vi "Send.vi"(8 "error in (no error)":errorcluster, 10 "Message":refnum<class "BaseMessage.lvclass">, 11 "QueueReader in":refnum<class "QueueReader.lvclass">) -> (0 "error out":errorcluster, 2 "Sent Message":refnum<class "BaseMessage.lvclass">, 3 "QueueReader out":refnum<class "QueueReader.lvclass">)   [LabVIEW 2013, in "QueueReader.lvclass"]
doc: "Send a message to the remote destination"
uses:
  QueueReader.lvclass
  Message/BaseMessage/BaseMessage.lvclass
  BaseReader/BaseReader.lvclass
  QueueReader.lvclass/QueueReader.ctl
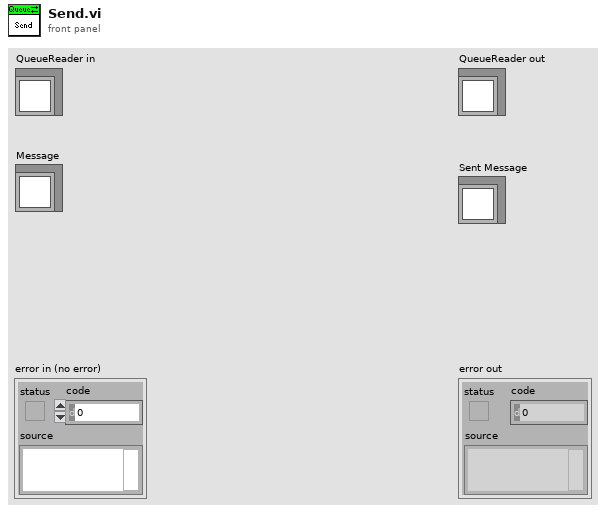
[diagram p1: front panel]
types:
  T1 = typedef "message_queue.ctl" = refnum<queue>
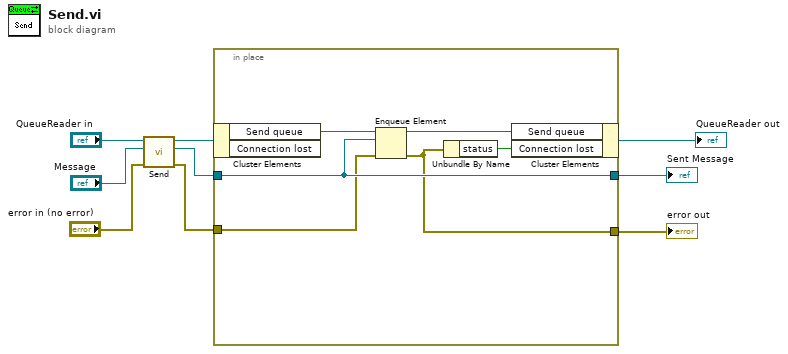
[diagram p0: block diagram]
diagram:
  n1 = call-parent "Send.vi"("error in (no error)"="error in (no error)", "Message"="Message", "BaseReader in"="QueueReader in") -> ("error out"=w1:errorcluster, "Sent Message"=w3:refnum<class "BaseMessage.lvclass">, "BaseReader out"=w5:refnum<class "QueueReader.lvclass">)  [unwired: 6 in]
  n2 = in-place "In Place Element Structure" {
    in-place-border: w3 -> [w15]
    in-place-border: [w15] -> w9
    in-place-border: w1 -> [w13]
    in-place-border: [w11] -> w7
    n3 = in-place-cluster #1(w5) -> ("Send queue"=w10:T1)  [unwired: 1 out]
    n4 = Enqueue Element(queue=w10, element=w15, error in (no error)=w13) -> (queue out=w14:T1, error out=w11:errorcluster)  [unwired: 1 in, 1 out]
    n5 = Unbundle By Name(w11) -> ("status"=w12:bool)
    n6 = in-place-cluster #1("Send queue"=w14, "Connection lost"=w12) -> (→"QueueReader out":refnum<class "QueueReader.lvclass">)
  }
  "error out" <- w7
  "Sent Message" <- w9
